vi "parse add search paths.vi"(8 "error in":errorcluster, 11 "message data":string) -> (0 "error out":errorcluster, 3 "paths":path[](array[path]))   [LabVIEW 2014, in "SMSLD TBD execution service.lvlib"]
uses:
  SMSLD TBD execution service.lvlib
  tokenized path.ctl
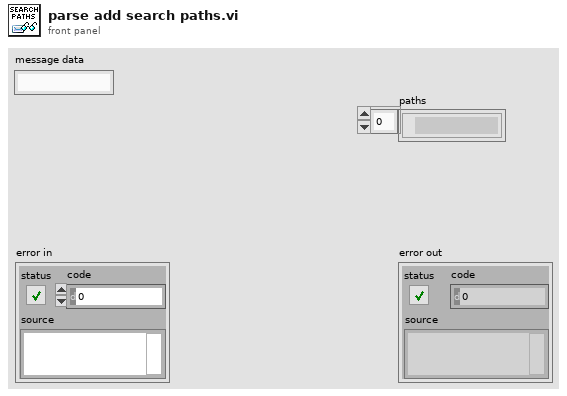
[diagram p1: front panel]
types:
  T1 = typedef "SMSLD TBD execution service.lvlib/tokenized path.ctl" = string[]
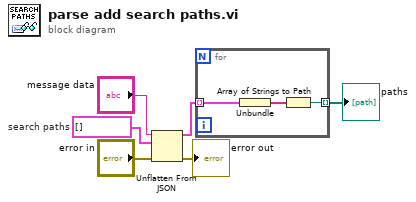
[diagram p0: block diagram]
diagram:
  w3 = cluster{"tokenized path":T1}[] []  # search paths
  n1 = Unflatten From JSON(JSON string="message data", type and defaults=w3, error in (no error)="error in") -> (value=w2:cluster{"tokenized path":T1}[], error out=→"error out":errorcluster)  [unwired: 4 in]
  n2 = for {
    tunnel: w2 -> [w9] mode=indexing
    tunnel: [w7] -> w1 mode=indexing
    n3 = Unbundle(w9) -> ("tokenized path"=w8:T1)
    n4 = Array of Strings to Path(0:w8) -> (2:w7:path)  [unwired: 1 in]
  }
  "paths" <- w1
